vi "Get Data Name from TD__ogtk.vi"(8 "error in (no error)":errorcluster, 10 "Type Descriptor":T1) -> (0 "error":errorcluster, 2 "name":string)   [LabVIEW 2012]
doc: "Returns the name of the data described by the type string input."
uses:
  <userlib>/_OpenG.lib/lvdata/lvdata.llb/Type Descriptor__ogtk.ctl
panel:
  # "[OpenG VI Tags] ***Do Not Remove***"
  # "Get Data Name from TD.vi\n\nReturns the name of the data described by the type string input.\n\nPlease visit http://www.OpenG.org to learn about the\nOpen Source LabVIEW software movement.\n\nNOTICE -- YOU MUST LEAVE THIS NOTICE IN PLACE.  PER THE TERMS OF THE LICENSE BELOW, YOU MAY SUBLICENSE THIS SOFTWARE \nIN ANY WAY THAT DOES NOT CONFLICT WITH THIS LICENSE.\n\n### BSD License (http://www.opensource.org/licenses/bsd-license.php) Begin ###\n \nCopyright (c) 2002, Jean-Pierre Drolet <drolet_jp@hotmail.com>\nCopyright (c) 2002-2006, Jim Kring <jim@jimkring.com>\n\nAll rights reserved.\n\nRedistribution and use in source and binary forms, with or without modification, are permitted provided that the following conditions are met:\n\n    * Redistributions of source code must retain the above copyright notice, this list of conditions and the following disclaimer.\n    * Redistributions in binary form must reproduce the above copyright notice, this list of conditions and the following disclaimer in the \n       documentation and/or other materials provided with the distribution.\n    * Neither the name of SciWare, James Kring, Inc., nor the names of its contributors may be used to endorse or promote products derived \n       from this software without specific prior written permission.\n\nTHIS SOFTWARE IS PROVIDED BY THE COPYRIGHT HOLDERS AND CONTRIBUTORS \"AS IS\" AND ANY EXPRESS OR IMPLIED WARRANTIES, \nINCLUDING, BUT NOT LIMITED TO, THE IMPLIED WARRANTIES OF MERCHANTABILITY AND FITNESS FOR A PARTICULAR PURPOSE ARE \nDISCLAIMED. IN NO EVENT SHALL THE COPYRIGHT OWNER OR CONTRIBUTORS BE LIABLE FOR ANY DIRECT, INDIRECT, INCIDENTAL,\n SPECIAL, EXEMPLARY, OR CONSEQUENTIAL DAMAGES (INCLUDING, BUT NOT LIMITED TO, PROCUREMENT OF SUBSTITUTE GOODS OR \nSERVICES; LOSS OF USE, DATA, OR PROFITS; OR BUSINESS INTERRUPTION) HOWEVER CAUSED AND ON ANY THEORY OF LIABILITY, \nWHETHER IN CONTRACT, STRICT LIABILITY, OR TORT (INCLUDING NEGLIGENCE OR OTHERWISE) ARISING IN ANY WAY OUT OF THE USE \nOF THIS SOFTWARE, EVEN IF ADVISED OF THE POSSIBILITY OF SUCH DAMAGE.\n\n### BSD License End ###"
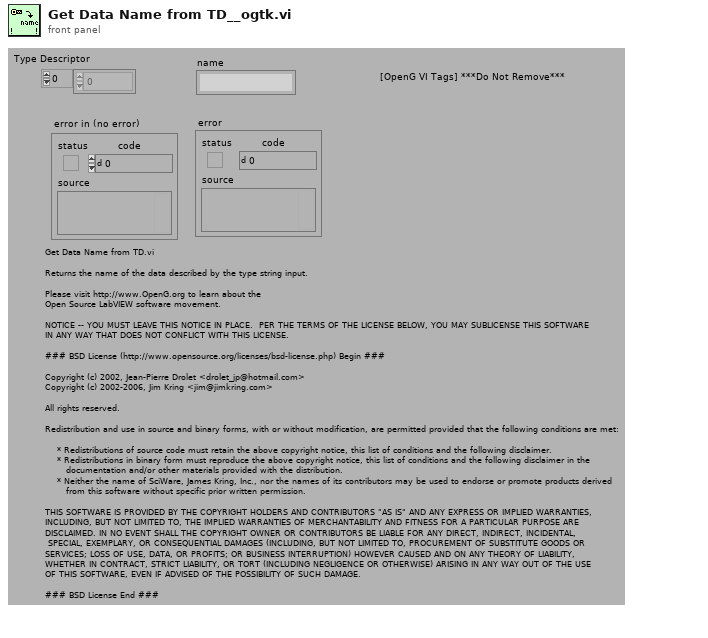
[diagram p1: front panel]
types:
  T1 = typedef "Type Descriptor__ogtk.ctl" = i16[]
  T2 = typedef "Type Descriptor Header__ogtk.ctl" = cluster{"length":u16, "private":u8, "type":T3, "# elements":u16}
  T3 = typedef "Type Descriptor Enumeration__ogtk.ctl" = enum8{"<Null>", "I8", "I16", "I32", "I64", "U8", "U16", "U32", "U64", "SGL", "DBL", "EXT", "CSG", "CDB", "CXT", "0x0F", "0x10", "0x11", "0x12", "0x13", "0x14", "Enum U8", "Enum U16", "Enum U32", "Enum U64", "SGL PQ", "DBL PQ", "EXT PQ", "CSG PQ", "CDB PQ", "CXT PQ", "0x1F", "0x20", "Boolean", "0x22", "0x23", "0x24", "0x25", "0x26", "0x27", "0x28", "0x29", "0x2A", "0x2B", "0x2C", "0x2D", "0x2E", "0x2F", "String", "0x31", "Path", "Pict", "0x34", "0x35", "0x36", "DAQ", "0x38", "0x39", "0x3A", "0x3B", "0x3C", "0x3D", "0x3E", "0x3F", "Array", "0x41", "0x42", "0x43", "0x44", "0x45", "0x46", "0x47", "0x48", "0x49", "0x4A", "0x4B", "0x4C", "0x4D", "0x4E", "0x4F", "Cluster", "0x51", "0x52", "Variant", "Waveform", "0x55", "0x56", "0x57", "0x58", "0x59", "0x5A", "0x5B", "0x5C", "0x5D", "0x5E", "0x5F", "0x60", "0x61", "0x62", "0x63", "0x64", "0x65", "0x66", "0x67", "0x68", "0x69", "0x6A", "0x6B", "0x6C", "0x6D", "0x6E", "0x6F", "Refnum"}
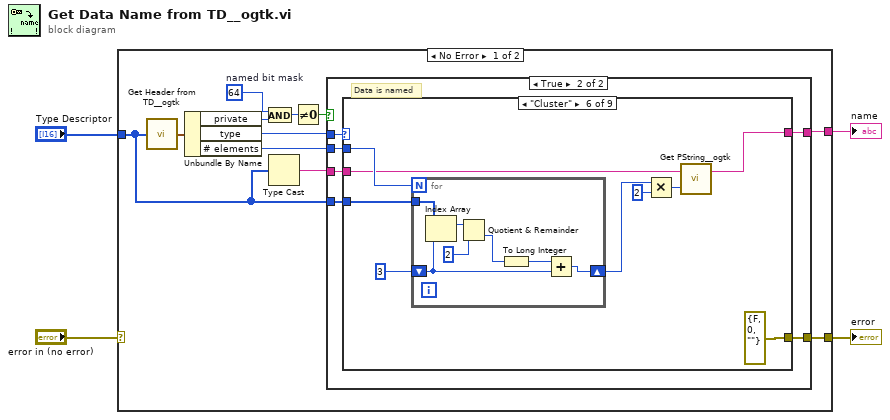
[diagram p0: block diagram]
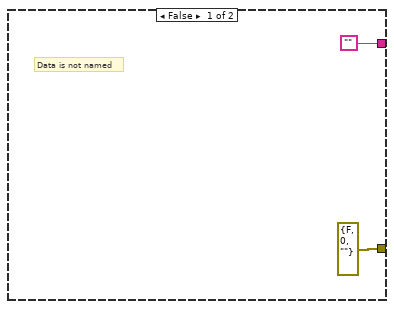
[diagram p2: hidden frame]
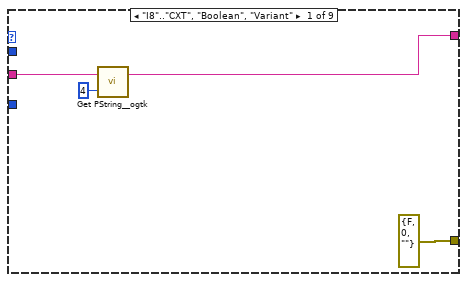
[diagram p3: hidden frame]
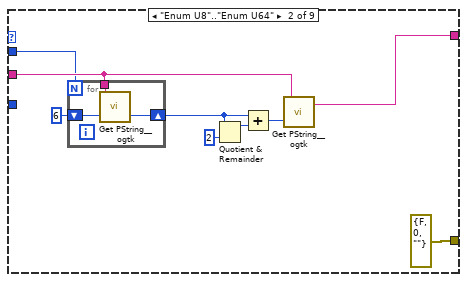
[diagram p4: hidden frame]
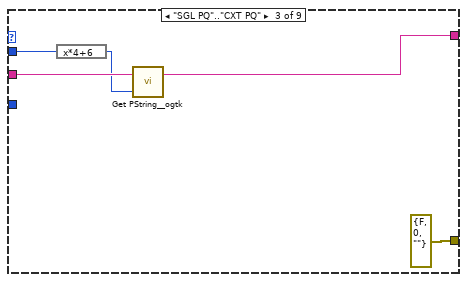
[diagram p5: hidden frame]
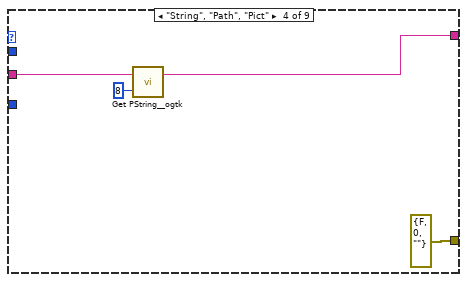
[diagram p6: hidden frame]
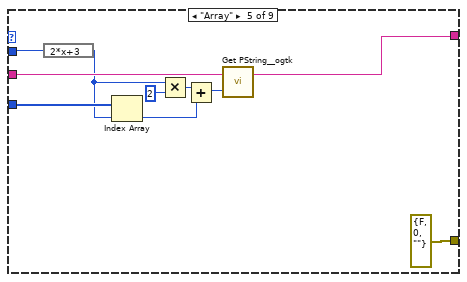
[diagram p7: hidden frame]
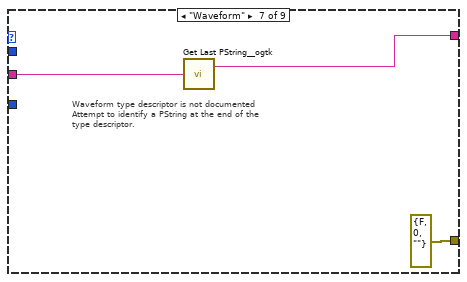
[diagram p8: hidden frame]
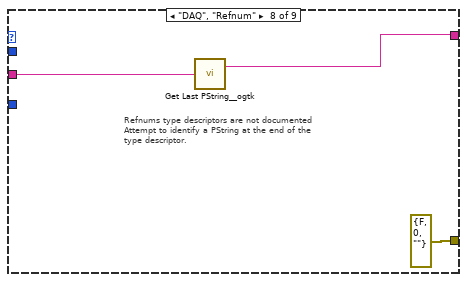
[diagram p9: hidden frame]
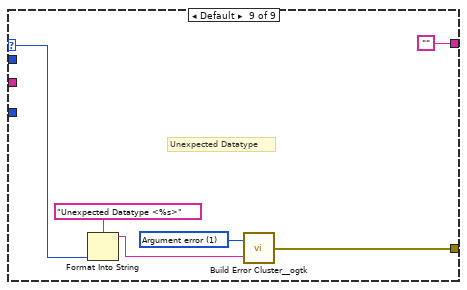
[diagram p10: hidden frame]
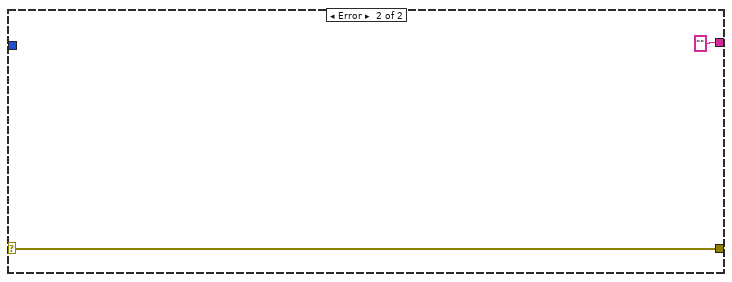
[diagram p11: hidden frame]
diagram:
  n1 = case shown="No Error" "error in (no error)" {
    selector: "error in (no error)" -> [_ w88]
    tunnel: "Type Descriptor" -> [w14 _]
    tunnel: [w11 "" ("Last PString")] -> w3
    tunnel: [w5 w88] -> w2
    frame No Error {
      w8 = u8 64  # named bit mask
      n2 = call <userlib>:"Get Header from TD__ogtk.vi"("Type Descriptor"=w14) -> ("Type Descriptor Header"=w15:T2)
      n3 = Unbundle By Name(w15) -> ("private"=w7:u8, "type"=w6:T3, "# elements"=w13:u16)
      n4 = And(x=w8, y=w7) -> (x .and. y?=w10:u8)
      n5 = Type Cast(x=w14) -> (*(type *) &x=w12:string)  [unwired: 1 in]
      n6 = Not Equal To 0?(x=w10) -> (x != 0?=w9:bool)
      n7 = case shown="True" w9 {
        tunnel: [errorcluster {"status"=FALSE, "code"=0, "source"=""} ("error out") w23] -> w5
        tunnel: w6 -> [_ w22]
        tunnel: w12 -> [_ w21]
        tunnel: ["" w20] -> w11
        tunnel: w13 -> [_ w19]
        tunnel: w14 -> [_ w18]
        frame False {
          # "Data is not named"
        }
        frame True {
          # "Data is named"
          n8 = case shown="\"Cluster\"" w22 {
            selector: w22 -> [_ _ _ _ _ _ _ _ w81]
            tunnel: [errorcluster {"status"=FALSE, "code"=0, "source"=""} ("error out") errorcluster {"status"=FALSE, "code"=0, "source"=""} ("error out") errorcluster {"status"=FALSE, "code"=0, "source"=""} ("error out") errorcluster {"status"=FALSE, "code"=0, "source"=""} ("error out") errorcluster {"status"=FALSE, "code"=0, "source"=""} ("error out") errorcluster {"status"=FALSE, "code"=0, "source"=""} ("error out") errorcluster {"status"=FALSE, "code"=0, "source"=""} ("error out") errorcluster {"status"=FALSE, "code"=0, "source"=""} ("error out") w86] -> w23
            tunnel: w21 -> [w26 w33 w43 w48 w55 w64 w76 w80 _]
            tunnel: [w24 w32 w41 w47 w54 w63 w75 w79 ""] -> w20
            tunnel: w19 -> [_ w30 w44 _ w57 w66 _ _ _]
            tunnel: w18 -> [_ _ _ _ w56 w65 _ _ _]
            frame "I8".."CXT", "Boolean", "Variant" {
              n9 = call <userlib>:"Get PString__ogtk.vi"("offset (0)"=4, "String"=w26) -> ("PString"=w24:string)  [unwired: 1 out]
            }
            frame "Enum U8".."Enum U64" {
              n10 = for {
                N: w30 -> [_]
                tunnel: w33 -> [w37]
                shift-right: [w38] -> w35
                shift-left: 6 -> [w39]
                n11 = call <userlib>:"Get PString__ogtk.vi"("offset (0)"=w39, "String"=w37) -> ("offset past PString"=w38:i32)  [unwired: 1 out]
              }
              n12 = Quotient & Remainder(x=w35, y=2) -> (x-y*floor(x/y)=w28:i32)  [unwired: 1 out]
              n13 = Add(x=w35, y=w28) -> (x+y=w34:i32)
              n14 = call <userlib>:"Get PString__ogtk.vi"("offset (0)"=w34, "String"=w33) -> ("PString"=w32:string)  [unwired: 1 out]
            }
            frame "SGL PQ".."CXT PQ" {
              n15 = expression code="x*4+6"(w44) -> (w42:u16)
              n16 = call <userlib>:"Get PString__ogtk.vi"("offset (0)"=w42, "String"=w43) -> ("PString"=w41:string)  [unwired: 1 out]
            }
            frame "String", "Path", "Pict" {
              n17 = call <userlib>:"Get PString__ogtk.vi"("offset (0)"=8, "String"=w48) -> ("PString"=w47:string)  [unwired: 1 out]
            }
            frame "Array" {
              n18 = expression code="2*x+3"(w57) -> (w53:u16)
              n19 = Index Array(array=w56, index=w53) -> (element=w50:i16)
              n20 = Multiply(x=w53, y=u16 2) -> (x*y=w51:u16)
              n21 = Add(x=w51, y=w50) -> (x+y=w49:u16)
              n22 = call <userlib>:"Get PString__ogtk.vi"("offset (0)"=w49, "String"=w55) -> ("PString"=w54:string)  [unwired: 1 out]
            }
            frame "Cluster" {
              n23 = for {
                N: w66 -> [_]
                shift-right: [w73] -> w61
                shift-left: 3 -> [w72]
                tunnel: w65 -> [w74]
                n24 = Index Array(array=w74, index=w72) -> (element=w70:i16)
                n25 = Quotient & Remainder(x=w70, y=i16 2) -> (floor(x/y)=w71:i16)  [unwired: 1 out]
                n26 = To Long Integer(number=w71) -> (32bit integer=w68:i32)
                n27 = Add(x=w68, y=w72) -> (x+y=w73:i32)
              }
              n28 = Multiply(x=w61, y=2) -> (x*y=w60:i32)
              n29 = call <userlib>:"Get PString__ogtk.vi"("offset (0)"=w60, "String"=w64) -> ("PString"=w63:string)  [unwired: 1 out]
            }
            frame "Waveform" {
              # "Waveform type descriptor is not documented\nAttempt to identify a PString at the end of the\ntype descriptor."
              n30 = call <userlib>:"Get Last PString__ogtk.vi"("String"=w76) -> ("Last PString"=w75:string)  [unwired: 1 out]
            }
            frame "DAQ", "Refnum" {
              # "Refnums type descriptors are not documented\nAttempt to identify a PString at the end of the\ntype descriptor."
              n31 = call <userlib>:"Get Last PString__ogtk.vi"("String"=w80) -> ("Last PString"=w79:string)  [unwired: 1 out]
            }
            frame Default {
              w85 = 1 items=["No error", "Argument error", "Memory is full", "Out of zone", "End of file", "File already open", "Generic file I/O error", "File not found", "File permission error", "Disk is full", "Duplicate path", "Too many files open", "System feature not enabled", "Resource file not found", "Cannot add resource", "Resource not found", "Image not found", "Image memory error", "Pen does not exist", "Config type invalid", "Config token not found", "Config parse error", "Config memory error", "Bad external code format", "Bad external code offset", "External code not present", "Null window", "Destroy window error", "Null menu", "Print aborted", "Bad print record", "Print driver error", "Windows error during printing", "Memory error during printing", "Print dialog error", "Generic print error", "Invalid device refnum", "Device not found", "Device parameter error", "Device unit error", "Cannot open device", "Device call aborted", "Generic error", "Cancelled by user", "Object ID too low", "Object ID too high", "Object not in heap", "Unknown heap", "Unknown object (invalid DefProc)", "Unknown object (DefProc not in table)", "Message out of range", "Invalid (null) method", "Unknown message", "Manager call not supported", "Bad address", "Network operation in progress", "Network operation timed out", "Connection is busy", "Network attribute not supported", "Network error", "Address in use", "System out of memory", "Connection aborted", "Connection refused", "Not connected", "Already connected", "Connection closed", "Initialization error (interapplication manager)", "Bad occurrence", "Wait on unbound occurrence handler", "Occurrence queue overflow", "Datalog type conflict", "Unused", "Unrecognized type (interapplication manager)", "Memory corrupt", "Failed to make temporary DLL", "Old CIN version", "Drag socket not found", "Failed to load drop-object", "Failed to register OLE object", "Failed to release OLE object", "Format specifier type mismatch", "Unknown format specifier", "Too few format specifiers", "Too many format specifiers", "Scan failed", "Newer CIN version", "Error converting to variant", "Runtime menu error", "Password tampered", "Variant attribute not found", "Incompatible variant data type", "Event data is not available", "Event Store is not present", "Occurrence is not found", "Event Queue is not created", "Event info is not available", "Refnum passed is NULL", "Error retrieving Class GUID", "Error retrieving CoClass GUID", "Error retrieving TypeLib GUID.", "Bad built application magic bytes.", "Specific driver is different from the specific driver associated with the Logical Name.", "There is no session opened to the class driver.", "Max Error", "MAX - Error with config objects", "MAX - Error loading configuration", "MAX - Group not supported"]
              # "Unexpected Datatype"
              n32 = Format Into String(format string="Unexpected Datatype <%s>" ("Format String"), w81) -> (resulting string=w82:string)  [unwired: 2 in, 1 out]
              n33 = call <userlib>:"Build Error Cluster__ogtk.vi"("String to Prepend to source (\"\")"=w82, "code"=w85) -> ("error out"=w86:errorcluster)
            }
          }
        }
      }
    }
    frame Error {
    }
  }
  "name" <- w3
  "error" <- w2
